vi "Main.vi"() -> ()   [LabVIEW 2014]
uses:
  <vilib>/LVH/AR Drone Toolkit/Decode NavData/Typedefs/NavData Demo.ctl
  <vilib>/LVH/AR Drone Toolkit/AR Drone.lvlib
panel:
  out "Video Stream":picture
  out "NavData Out":T1
  out "Control cluster":T2 {"Roll" scale=-1.0..1.0; "Pitch" scale=-1.0..1.0; "Vertical Speed" scale=-1.0..1.0; "Yaw Speed" scale=-1.0..1.0}
  in  "Emergency Landing":bool
  in  "Takeoff/Land":bool
  in  "Setup Parameters":T3={"Drone IP address"="192.168.1.1", "Home IP address"="192.168.1.2", "Flight Mode"=enum."INDOOR MODE", "Mounted Hull"=enum."INDOOR HULL", "Video Camera"=2, "Max Altitude (m)"=3.0, "Max Pitch and Roll Angle (deg)"=10.0, "Max Vertical Speed (m/s)"=0.7, "Max Yaw Speed (deg/s)"=100.0} {"Video Camera" items=["Bottom Camera"=1, "Front Camera"=0, "Front in Bottom"=3, "Bottom in Front"=2]}
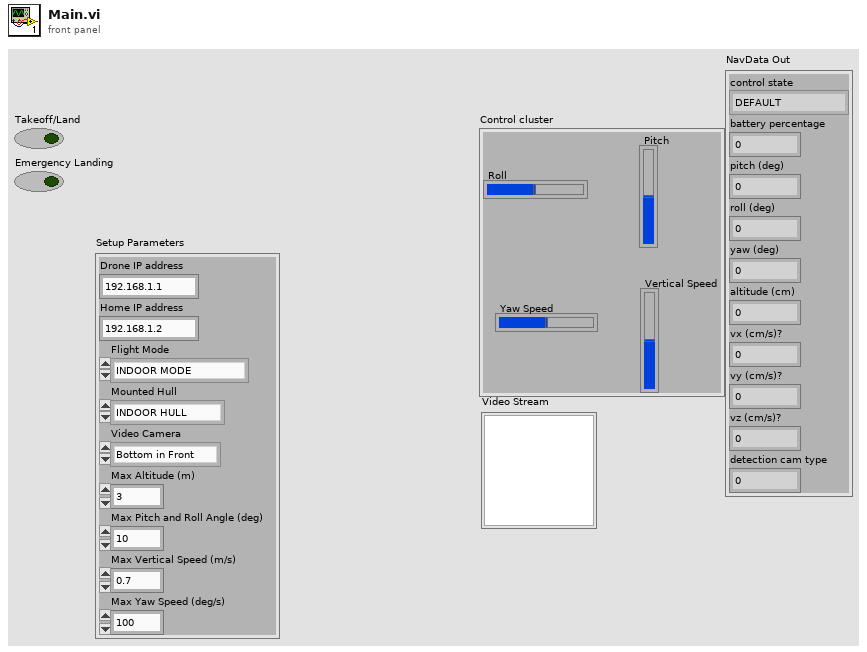
[diagram p1: front panel]
types:
  T1 = typedef "AR Drone.lvlib/NavData Demo.ctl" = cluster{"control state":enum32{"DEFAULT", "INIT", "LANDING", "FLYING", "HOVERING", "TEST", "TRANS_TAKEOFF", "TRANS_GOTOFIX", "TRANS_LANDING"}, "battery percentage":u32, "pitch (deg)":sgl, "roll (deg)":sgl, "yaw (deg)":sgl, "altitude (cm)":u32, "vx (cm/s)?":sgl, "vy (cm/s)?":sgl, "vz (cm/s)?":sgl, "detection cam type":u32}
  T2 = cluster{"Roll":dbl, "Pitch":dbl, "Vertical Speed":dbl, "Yaw Speed":dbl}
  T3 = cluster{"Drone IP address":string, "Home IP address":string, "Flight Mode":enum8{"OUTDOOR MODE", "INDOOR MODE"}, "Mounted Hull":enum8{"OUTDOOR HULL", "INDOOR HULL"}, "Video Camera":u8, "Max Altitude (m)":sgl, "Max Pitch and Roll Angle (deg)":sgl, "Max Vertical Speed (m/s)":sgl, "Max Yaw Speed (deg/s)":sgl}
  T4 = typedef "AR Drone.lvlib/AR Drone Resource.ctl" = cluster{"UDP Control Connection":refnum<k16>, "UDP NavData Connection":refnum<k16>, "UDP Video Connection (Drone 1.0)":refnum<k16>, "TCP Video Connection (Drone 2.0)":refnum<k5>, "TCP Control Port Connection":refnum<k5>, "Drone IP address":string, "Drone Command Port":u16, "Drone NavData Port":u16, "Drone Vid Stream Port":u16, "Drone TCP Control Port":u16, "Home IP address":string, "Home Command Port":u16, "Home NavData Port":u16, "Home Vid Stream Port":u16, "Drone Version":i32, "Drone Index":i32, "Command Sequence":i32}
  T5 = cluster{"Hover":bool, bool, "Emergency Landing":bool, "button 4":bool, "button 5":bool, "button 6":bool, "button 7":bool, "button 8":bool}
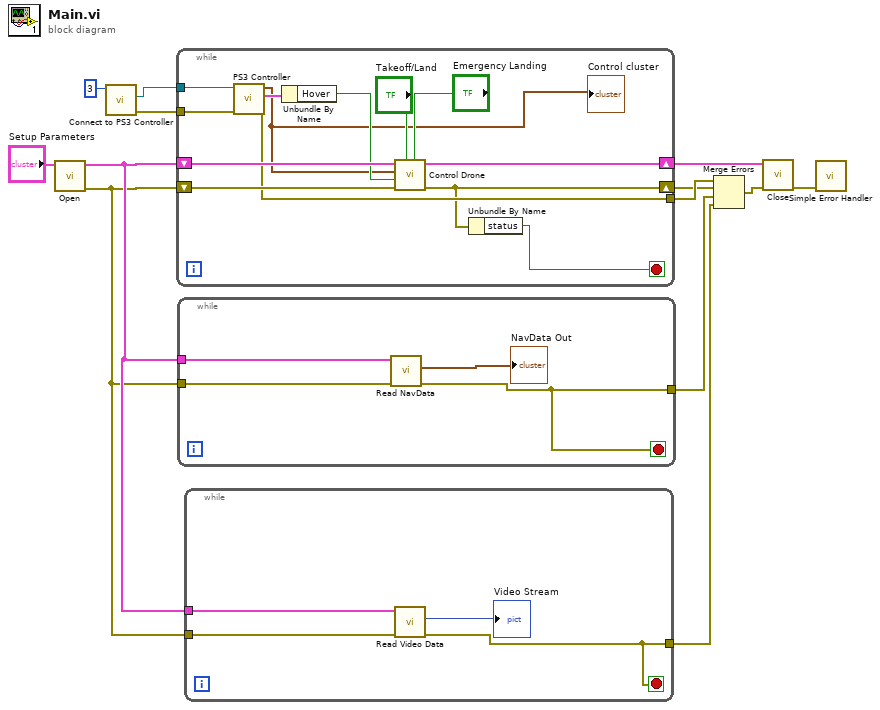
[diagram p0: block diagram]
diagram:
  n1 = call <vilib>:"Open.vi"("Setup Parameters"="Setup Parameters") -> ("error out"=w7:errorcluster, "AR Drone Resource"=w8:T4)  [unwired: 9 in]
  n2 = call "Connect to PS3 Controller.vi"("device ID"=3) -> ("error out"=w10:errorcluster, "device ID 2"=w11:refnum<k1>)  [unwired: 7 in, 1 out]
  n3 = while {
    shift-right: [w25] -> w13
    shift-left: w8 -> [w26]
    shift-right: [w15] -> w5
    shift-left: w7 -> [w24]
    tunnel: w11 -> [w23]
    tunnel: w10 -> [w22]
    tunnel: [w16] -> w6
    stop <- w14 stop-if-true
    n4 = call "PS3 Controller.vi"("error in (no error)"=w22, "device ID"=w23) -> ("error out"=w16:errorcluster, "Buttons"=w21:T5, "Control cluster"=w17:T2)  [unwired: 6 in, 1 out]
    "Control cluster" <- w17
    n5 = Unbundle By Name(w21) -> ("Hover"=w20:bool)
    n6 = call <vilib>:"Control Drone.vi"("Emergency Landing"="Emergency Landing", "Takeoff/Land"="Takeoff/Land", "error in (no error)"=w24, "Hover"=w20, "Control Cluster"=w17, "AR Drone Resource"=w26) -> ("error out"=w15:errorcluster, "AR Drone Resource Out"=w25:T4)  [unwired: 4 in]
    n7 = Unbundle By Name(w15) -> ("status"=w14:bool)
  }
  n8 = while {
    tunnel: w8 -> [w30]
    tunnel: w7 -> [w29]
    tunnel: [w27] -> w4
    stop <- w27 stop-if-true
    n9 = call <vilib>:"Read NavData.vi"("error in (no error)"=w29, "AR Drone Resource"=w30) -> ("error out"=w27:errorcluster, "NavData Out"=→"NavData Out":T1)  [unwired: 7 in, 1 out]
  }
  n10 = while {
    tunnel: w8 -> [w34]
    tunnel: w7 -> [w33]
    tunnel: [w31] -> w3
    stop <- w31 stop-if-true
    n11 = call <vilib>:"Read Video Data.vi"("error in (no error)"=w33, "AR Drone Resource"=w34) -> ("error out"=w31:errorcluster, "Video Stream"=→"Video Stream":picture)  [unwired: 7 in, 1 out]
  }
  n12 = Merge Errors(w6, w5, w4, w3) -> (w2:errorcluster)
  n13 = call <vilib>:"Close.vi"("error in (no error)"=w2, "AR Drone Resource"=w13) -> ("error out"=w1:errorcluster)  [unwired: 9 in]
  n14 = call <vilib>:"Simple Error Handler.vi"("error in (no error)"=w1) -> ()  [unwired: 4 in, 5 out]
